vi "Main_Decode_V3.vi"(0 "GEA2 Reference In":refnum<k24>, 1 "GEA Inputs":T7={"Source"=228, "Destination"=0} {"Destination" format="%.0x"; "Source" format="%.0x"}, 5 "Error In":errorcluster) -> (7 "Fault Set?":bool[](array[boolean]), 9 "Fault Table Status":T4[](array[typedef]), 10 "Major Version":u8, 11 "Raw Snap Data":string[][](array[string]), 12 "Minor Version":u8, 13 "Fault Table Entries":T5[][](array[typedef]), 14 "GEA2 Reference Out":refnum<k24>, 15 "Diagnostic Entity Manifest":T2[](array[typedef]), 16 "SnapShot ERD List":T3[][](array[typedef]) {"ERD Number" format="%.0x"}, 17 "Fault Sequence Status":T4[](array[typedef]), 18 "Fault Sequence Entries":T6[][](array[typedef]), 19 "Error Out":errorcluster)   [LabVIEW 2023]
uses:
  LabVIEW GEA2 Toolkit/GEA3/type defs/Source_Destination.ctl
  D:/Common/LabVIEW GEA2 Toolkit/source/GEA3 DLL Source/GeaCommunication.dll
  LabVIEW GEA2 Toolkit/source/GEA3 DLL Source/GeaCommunication.dll
  Type Defs/Diag_FaultSeqEntry.ctl
  Type Defs/Diag_FaultTableStatus.ctl
  Type Defs/Diag_FaultTableEntry.ctl
  Type Defs/Diag_EntityManifestType.ctl
  LabVIEW GEA2 Toolkit/GEA3/type defs/ERD Read Data In.ctl
  LabVIEW GEA2 Toolkit/GEA3/library/GEA2_Toolkit.lvlib
panel:
  in  "Tab Control":T1(tab)
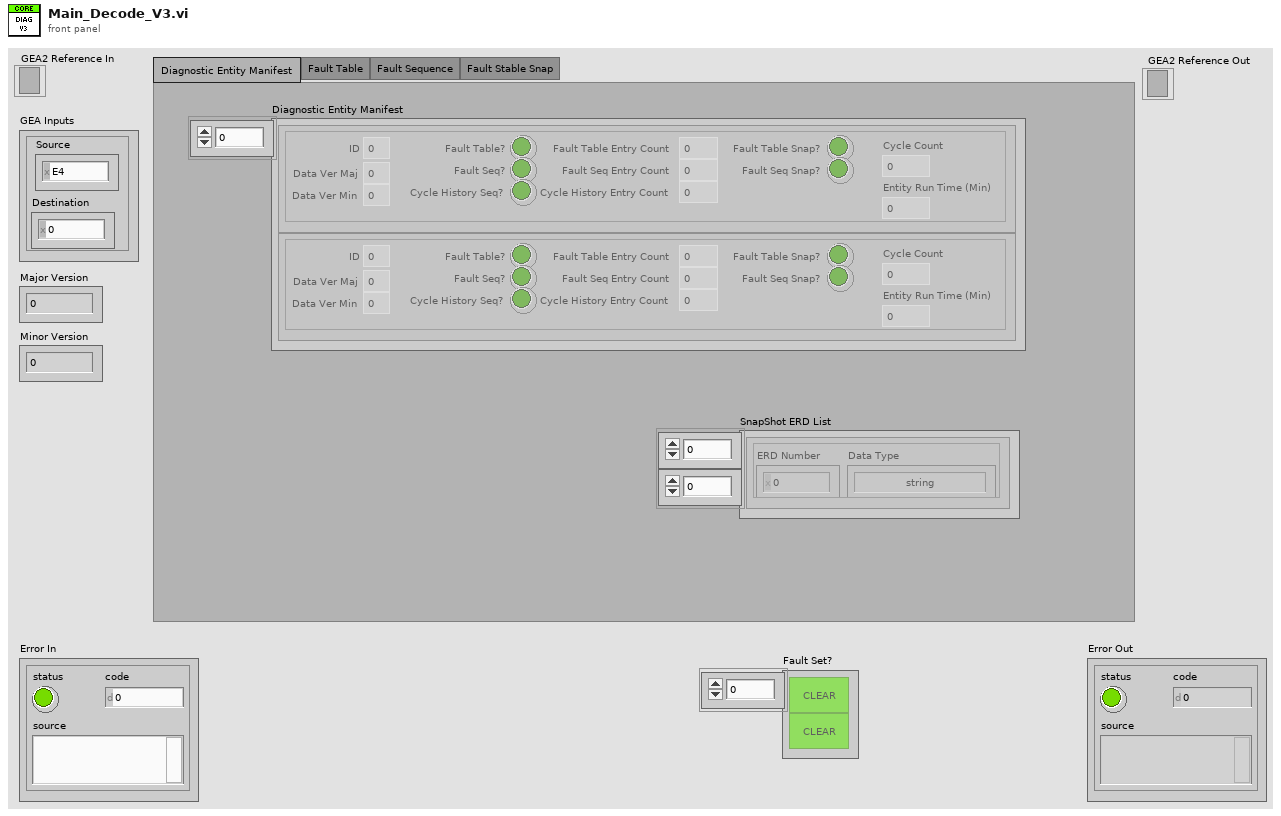
[diagram p1: front panel]
types:
  T1 = enum32{"Diagnostic Entity Manifest ", "Fault Table", "Fault Sequence", "Fault Stable Snap"}
  T2 = typedef "Diag_EntityManifestType.ctl" = cluster{"ID":u8, "Data Ver Maj":u8, "Data Ver Min":u8, "Fault Table?":bool, "Fault Table Snap?":bool, "Fault Seq?":bool, "Fault Seq Snap?":bool, "Cycle History Seq?":bool, "Fault Table Entry Count":u16, "Fault Seq Entry Count":u16, "Cycle History Entry Count":u16, "Cycle Count":u32, "Entity Run Time (Min)":u32}
  T3 = typedef "ERD Read Data In.ctl" = cluster{"ERD Number":u16, "Data Type":enum16{"string", "boolean", "uint8_t", "uint16_t", "uint32_t", "uint64_t", "int8_t", "int16_t", "int32_t", "int64_t"}}
  T4 = typedef "Diag_FaultTableStatus.ctl" = cluster{"Cur Index":u16, "Count":u16, "Ov Cnt":u16}
  T5 = typedef "Diag_FaultTableEntry.ctl" = cluster{"Cycle #":u32, "Time":u32, "F Code":string, "F Count":u16, "F Active":bool}
  T6 = typedef "Diag_FaultSeqEntry.ctl" = cluster{"Cycle #":u32, "Time":u32, "F Code":string, "F Active":bool}
  T7 = typedef "Source_Destination.ctl" = cluster{"Source":u8, "Destination":u8}
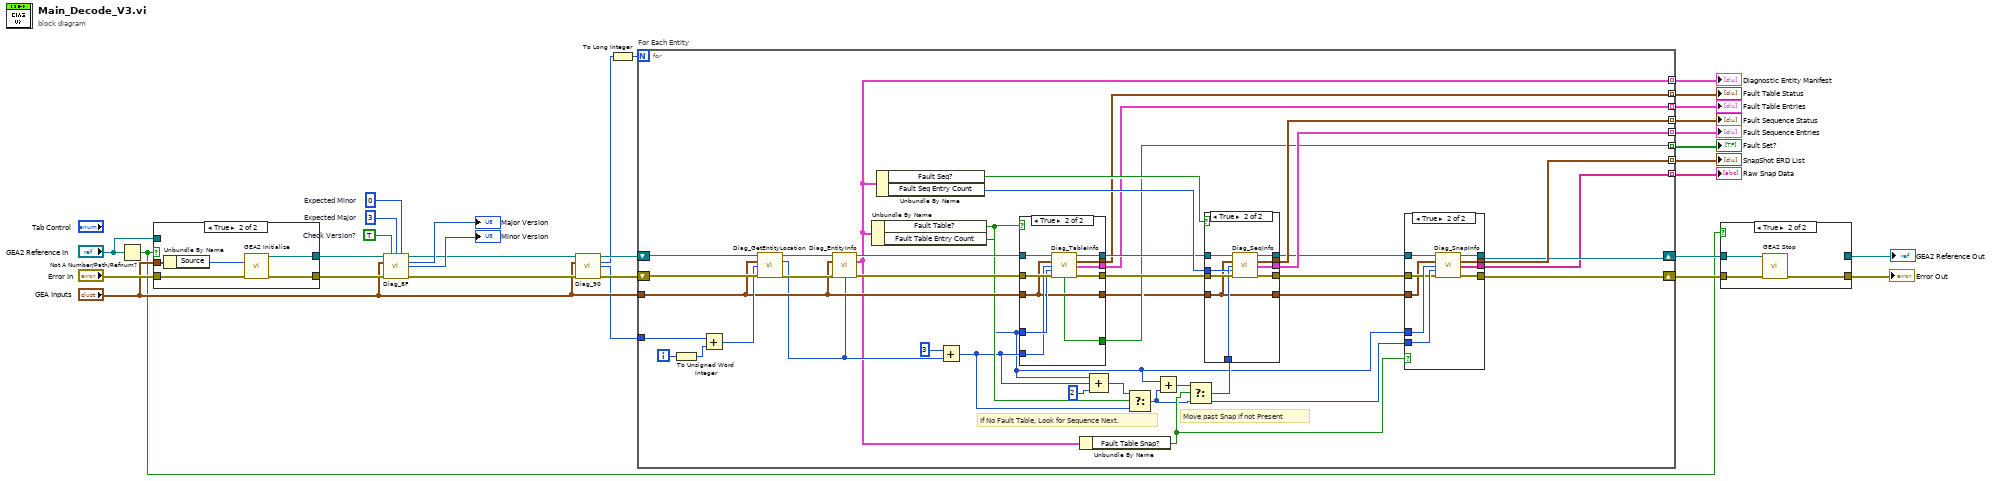
[diagram p0: block diagram]
diagram:
  w20 = u8 0  # Expected Minor
  w21 = u8 3  # Expected Major
  w24 = TRUE  # Check Version?
  n1 = Not A Number/Path/Refnum?(number/path/refnum="GEA2 Reference In") -> (NaN/Path/Refnum?=w11:bool)
  n2 = case shown="True" w11 {
    tunnel: "Error In" -> [w31 w37]
    tunnel: "GEA Inputs" -> [_ w35]
    tunnel: [w31 w34] -> w26
    tunnel: [w32 w33] -> w25
    tunnel: "GEA2 Reference In" -> [w32 _]
    frame False {
    }
    frame True {
      n3 = Unbundle By Name(w35) -> ("Source"=w36:u8)
      n4 = call "GEA2 Initialize.vi"("Source Address"=w36, "error in"=w37) -> ("GEA2 Reference Out"=w33:refnum<k24>, "error out"=w34:errorcluster)  [unwired: 10 in, 2 out]
    }
  }
  n5 = call "Diag_8F.vi"("GEA2 Reference In"=w25, "Check Version?"=w24, "Expected Major"=w21, "Expected Minor"=w20, "GEA Inputs"="GEA Inputs", "Error In"=w26) -> ("GEA2 Reference Out"=w19:refnum<k24>, "Major Version"=→"Major Version":u8, "Minor Version"=→"Minor Version":u8, "Error Out"=w28:errorcluster)  [unwired: 6 in]
  n6 = call "Diag_90.vi"("GEA2 Reference In"=w19, "GEA Inputs"="GEA Inputs", "Error In"=w28) -> ("GEA2 Reference Out"=w18:refnum<k24>, "Diagnostics Entity Count"=w6:u8, "Diagnostic Entity Map Location"=w16:u16, "Error Out"=w27:errorcluster)  [unwired: 9 in]
  n7 = To Long Integer(number=w6) -> (32bit integer=w5:i32)
  n8 = for "For Each Entity" {
    N: w5 -> [_]
    shift-right: [w42] -> w12
    shift-left: w18 -> [w73]
    tunnel: w16 -> [w77]
    shift-right: [w40] -> w15
    shift-left: w27 -> [w74]
    tunnel: "GEA Inputs" -> [w67]
    tunnel: [w54] -> w7 mode=indexing
    tunnel: [w53] -> w8 mode=indexing
    tunnel: [w52] -> w9 mode=indexing
    tunnel: [w51] -> w10 mode=indexing
    tunnel: [w50] -> w4 mode=indexing
    tunnel: [w49] -> w3 mode=indexing
    tunnel: [w43] -> w2 mode=indexing
    tunnel: [w38] -> w1 mode=indexing
    i -> [w76]
    # "Move past Snap if not Present"
    # "If No Fault Table, Look for Sequence Next."
    n9 = To Unsigned Word Integer(number=w76) -> (unsigned 16bit integer=w75:u16)
    n10 = Add(x=w77, y=w75) -> (x+y=w72:u16)
    n11 = call "Diag_GetEntityLocation.vi"("GEA2 Reference In"=w73, "GEA Inputs"=w67, "ERD Number from ERD 0x90"=w72, "Error In"=w74) -> ("GEA2 Reference Out"=w71:refnum<k24>, "Diagnostics Entity Location"=w64:u16, "Error Out"=w70:errorcluster)  [unwired: 9 in]
    n12 = call "Diag_EntityInfo.vi"("GEA2 Reference In"=w71, "GEA Inputs"=w67, "Error In"=w70, "Entity Location"=w64) -> ("GEA2 Reference Out"=w69:refnum<k24>, "Diagnostic Entity Manifest"=w50:T2, "Error Out"=w68:errorcluster)  [unwired: 9 in]
    n13 = Unbundle By Name(w50) -> ("Fault Table?"=w65:bool, "Fault Table Entry Count"=w47:u16)
    n14 = Unbundle By Name(w50) -> ("Fault Seq?"=w57:bool, "Fault Seq Entry Count"=w56:u16)
    n15 = Add(x=u16 3, y=w64) -> (x+y=w61:u16)
    n16 = case shown="True" w65 {
      tunnel: w69 -> [w103 w113]
      tunnel: w68 -> [w102 w112]
      tunnel: w47 -> [_ w111]
      tunnel: w67 -> [w101 w105]
      tunnel: w61 -> [_ w110]
      tunnel: [_ w109] -> w54
      tunnel: [_ w108] -> w53
      tunnel: [w103 w107] -> w55
      tunnel: [w102 w106] -> w59
      tunnel: [w101 w105] -> w45
      tunnel: [_ w104] -> w49
      frame False {
      }
      frame True {
        n17 = call "Diag_TableInfo.vi"("GEA2 Reference In"=w113, "GEA Inputs"=w105, "Table Status Location"=w110, "Table Entry Count"=w111, "Error In"=w112) -> ("GEA2 Reference Out"=w107:refnum<k24>, "Fault Table Status"=w109:T4, "Fault Table Entries"=w108:T5[], "Fault Set?"=w104:bool, "Error Out"=w106:errorcluster)  [unwired: 6 in]
      }
    }
    n18 = Unbundle By Name(w50) -> ("Fault Table Snap?"=w48:bool)
    n19 = Compound Arithmetic op=ADD(w47, w61, u16 2 ("value")) -> (w62:u16)
    n20 = Select(t=w62, s=w65, f=w61) -> (s? t:f=w44:u16)
    n21 = Add(x=w47, y=w44) -> (x+y=w60:u16)
    n22 = Select(t=w60, s=w48, f=w44) -> (s? t:f=w58:u16)
    n23 = case shown="True" w57 {
      tunnel: w59 -> [w91 w100]
      tunnel: w58 -> [_ w99]
      tunnel: w56 -> [_ w98]
      tunnel: w55 -> [w90 w97]
      tunnel: [w90 w96] -> w46
      tunnel: [w91 w95] -> w41
      tunnel: w45 -> [w89 w92]
      tunnel: [_ w94] -> w52
      tunnel: [_ w93] -> w51
      tunnel: [w89 w92] -> w39
      frame False {
      }
      frame True {
        n24 = call "Diag_SeqInfo.vi"("GEA2 Reference In"=w97, "GEA Inputs"=w92, "Seq Status Location"=w99, "Seq Entry Count"=w98, "Error In"=w100) -> ("GEA2 Reference Out"=w96:refnum<k24>, "Fault Seq Status"=w94:T4, "Fault Sequence Entries"=w93:T6[], "Error Out"=w95:errorcluster)  [unwired: 7 in]
      }
    }
    n25 = case shown="True" w48 {
      tunnel: w47 -> [_ w88]
      tunnel: w46 -> [w79 w87]
      tunnel: w44 -> [_ w86]
      tunnel: [_ w85] -> w43
      tunnel: [w79 w84] -> w42
      tunnel: w41 -> [w78 w83]
      tunnel: [w78 w82] -> w40
      tunnel: w39 -> [_ w81]
      tunnel: [_ w80] -> w38
      frame False {
      }
      frame True {
        n26 = call "Diag_SnapInfo.vi"("GEA2 Reference In"=w87, "GEA Inputs"=w81, "Table Entry Count"=w88, "Table Status Location"=w86, "Error In"=w83) -> ("GEA2 Reference Out"=w84:refnum<k24>, "Snap Location"=w85:T3[], "Raw Snap Data"=w80:string[], "Error Out"=w82:errorcluster)  [unwired: 7 in]
      }
    }
  }
  "Fault Sequence Entries" <- w10
  "Fault Sequence Status" <- w9
  "Fault Table Entries" <- w8
  "Fault Table Status" <- w7
  "Diagnostic Entity Manifest" <- w4
  "Fault Set?" <- w3
  "SnapShot ERD List" <- w2
  "Raw Snap Data" <- w1
  n27 = case shown="True" w11 {
    tunnel: w15 -> [w114 w118]
    tunnel: [w114 w117] -> w14
    tunnel: [w115 _] -> w13
    tunnel: w12 -> [w115 w116]
    frame False {
    }
    frame True {
      n28 = call "GEA2 Stop.vi"("GEA2 Reference In"=w116, "Error In"=w118) -> ("Error Out"=w117:errorcluster)  [unwired: 13 in]
    }
  }
  "Error Out" <- w14
  "GEA2 Reference Out" <- w13
